vi "SetParamWaveType.vi"(1 "ParamWaveType":u16(ring) items=["Sine", "Pulse", "Sweep", "Sinc", "Exponential", "Prbs", "Square", "Multitone"], 3 "error in (no error)":errorcluster, 4 "ParamWave Name":string, 5 "VISA resource name":refnum<visa-resource-name>) -> (0 "error out":errorcluster, 2 "VISA resource name out":refnum<visa-resource-name>)   [LabVIEW 2020, in "Active Technologies AWG3000.lvlib"]
uses:
  Active Technologies AWG3000.lvlib
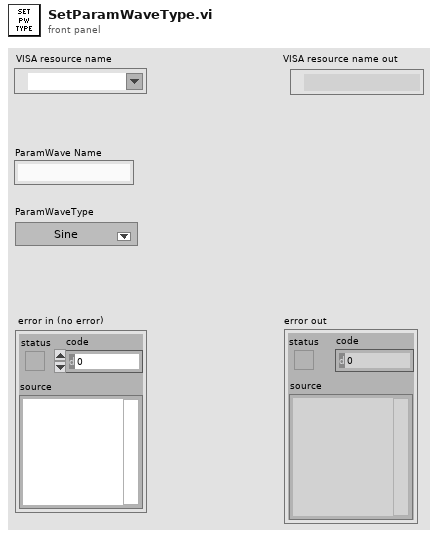
[diagram p1: front panel]
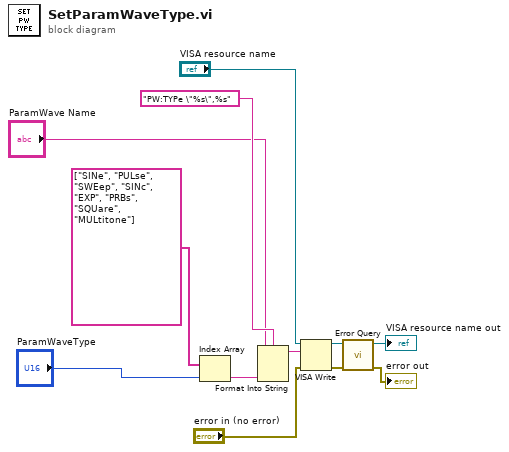
[diagram p0: block diagram]
diagram:
  n1 = Index Array(array=string[] ["SINe", "PULse", "SWEep", "SINc", "EXP", "PRBs", "SQUare", "MULtitone"], index="ParamWaveType") -> (element=w3:string)
  n2 = Format Into String(format string="PW:TYPe \"%s\",%s" ("write buffer"), "ParamWave Name", w3) -> (resulting string=w9:string)  [unwired: 2 in, 1 out]
  n3 = VISA Write(VISA resource name="VISA resource name", write buffer=w9, error in (no error)="error in (no error)") -> (VISA resource name out=w8:refnum<visa-resource-name>, error out=w7:errorcluster)  [unwired: 1 out]
  n4 = call "Error Query.vi"("error in (no error)"=w7, "VISA resource name"=w8) -> ("error out"=→"error out":errorcluster, "VISA resource name out"=→"VISA resource name out":refnum<visa-resource-name>)  [unwired: 6 in, 2 out]
